vi "Integer Matrix.vi"() -> (0 "error out":errorcluster, 3 "Passed?":bool)   [LabVIEW 2009]
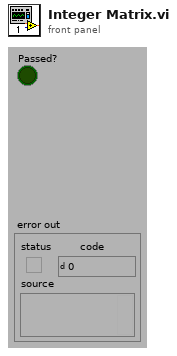
[diagram p1: front panel]
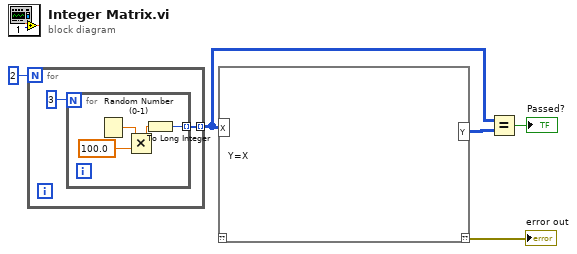
[diagram p0: block diagram]
diagram:
  n1 = for {
    N: 2 -> [_]
    tunnel: [w6] -> w3 mode=indexing
    n2 = for {
      N: 3 -> [_]
      tunnel: [w11] -> w6 mode=indexing
      n3 = Random Number (0-1)() -> (number: 0 to 1=w10:dbl)
      n4 = Multiply(x=w10, y=100.0) -> (x*y=w8:dbl)
      n5 = To Long Integer(number=w8) -> (32bit integer=w11:i32)
    }
  }
  n6 = script code="Y=X"("X"=w3) -> ("??"=→"error out":errorcluster, "Y"=w2:i32[][])  [unwired: 1 in]
  n7 = Equal?(x=w3, y=w2) -> (x = y?=→"Passed?":bool)
